vi "SendTriggerCAN.vi"(8 "error in (no error)":errorcluster, 11 "interface object in":refnum<k20>) -> (0 "error out":errorcluster, 3 "interface object out":refnum<k20>)   [LabVIEW 2014]
uses:
  <vilib>/RioEmbeddedCAN/RioEmbeddedCAN.llb/CANFrameControl.ctl
  Global Data.vi
  <vilib>/RioEmbeddedCAN/RioEmbeddedCAN.llb/CANWaitTransmitComplete.vi
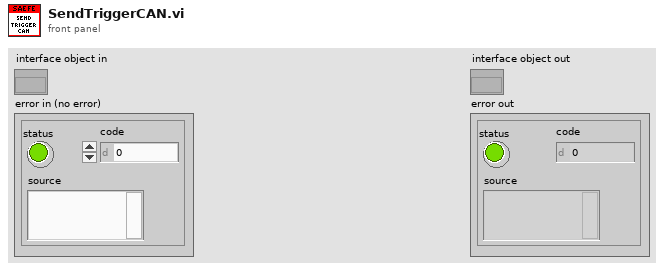
[diagram p1: front panel]
types:
  T1 = typedef "CANFrameControl.ctl" = cluster{"identifier":u32, "extended?":bool, "type":u8, "payload":u8[]}
  T2 = typedef "FPGA Telemetry.ctl" = cluster{"CPU Load":cluster{"Total (%)":dbl, "Time Critical (%)":dbl, "Timed Structures (%)":dbl, "High (%)":dbl, "Above Normal (%)":dbl, "Normal (%)":dbl, "Background (%)":dbl, "Idle (%)":dbl, "ISR (%)":dbl}, "SVehicleStatus":cluster{"BMS Status":T3, "MC Status":T3, "Shutdown Status":T3, "sbRIO Status":T3, "Vehicle Status":T3, "Shutdown State":enum16{"NI.SC.Initial", "NI.SC.History", "NI.SC.ShallowHistory", "NI.SC.Terminal", "Coolant Pump Started/AIR's On", "AIRs On", "Precharge", "TSMS Off"}, "AIR Status":T6, "Remote Return to Pits":bool, "Reason for Shutdown":T7, "MC State Machine Status":enum16{"NI.SC.Initial", "NI.SC.History", "NI.SC.ShallowHistory", "NI.SC.Terminal", "Broadcast Diag", "Let Current Drop then Disable AIR's", "Enabled", "Disabled"}}, "iPhone HF Data":cluster{"gXiPhone":dbl, "gYiPhone":dbl, "gZiPhone":dbl, "nYawXiPhone":dbl, "nYawYiPhone":dbl, "nYawZiPhone":dbl}, "iPhone LF Data":cluster{"nLatiPhone":dbl, "nLongiPhone":dbl, "nGPSiPhone":dbl}, "stop":bool, "VSupplyOffset":fxp<+,12,4>, "VsbRIOSupply":fxp<+/-,25,6>, "bFPGALED":bool, "TSBRIO":fxp<+/-,33,17>, "rTPS2Unscaled":fxp<+/-,16,1>, "rTPS1Unscaled":fxp<+/-,16,1>, "bTPSConsistent":bool, "bTPSInRange":bool, "rThrottle":fxp<+/-,33,22>, "VTPS2":fxp<+/-,24,5>, "rTPS2":fxp<+/-,31,22>, "VTPS1":fxp<+/-,24,5>, "rTPS1":fxp<+/-,31,22>, "rTPS2Max":fxp<+,16,4>, "rTPS2Min":fxp<+,16,4>, "rTPS1Max":fxp<+,16,4>, "rTPS1Min":fxp<+,16,4>, "bCoolantPumpEnable":bool, "bRTDSEnable":bool, "bTSMSInStatus":bool, "bPosAIREnable":bool, "bBMSOK":bool, "bIMDOK":bool, "bBSPDOK":bool, "bSBRIOOK2":bool, "bSBRIOOK1":bool, "bTSMSOutStatus":bool, "eGreenDash":T8, "eYellowDash":T8, "eRedDash":T8, "bMotorControllerEnable":bool, "tCurrentLap":u32, "bNewLap":bool, "tLastLap":u32, "tLapMin":u32, "V5VSupply":fxp<+/-,24,5>, "bWheelRL":bool, "bWheelRR":bool, "bWheelFR":bool, "bWheelFL":bool, "VBrakePressureR":fxp<+/-,24,5>, "VBrakePressureF":fxp<+/-,24,5>, "bWheelRRStopped":bool, "bWheelRLStopped":bool, "bWheelFRStopped":bool, "bWheelFLStopped":bool, "tWheelRLPeriod":u32, "tWheelRRPeriod":u32, "tWheelFRPeriod":u32, "tWheelFLPeriod":u32, "bBrakeLight":bool, "VShockRR":fxp<+/-,24,5>, "VShockRL":fxp<+/-,24,5>, "VShockFR":fxp<+/-,24,5>, "VShockFL":fxp<+/-,24,5>, "IHighCurrent":fxp<+/-,24,15>, "ILowCurrent":fxp<+/-,24,15>, "pBrakeR":fxp<+,26,13>, "pBrakeF":fxp<+,26,13>, "bHighCurrentOK":bool, "bLowCurrentOK":bool, "bBrakeROK":bool, "bBrakeFOK":bool, "VSteerWheelMiddle":fxp<+/-,26,5>, "aSteerWheel":fxp<+/-,31,13>, "nWheelFL":fxp<+/-,32,16>, "nWheelFR":fxp<+/-,32,16>, "nWheelRL":fxp<+/-,32,16>, "nWheelRR":fxp<+/-,32,16>, "ADXL345 Output":T9, "Tire Diameter(m)":fxp<+,16,1>, "vWheelRR":fxp<+/-,32,18>, "vWheelRL":fxp<+/-,32,18>, "vWheelFR":fxp<+/-,32,18>, "vWheelFL":fxp<+/-,32,18>, "vWheelLowest":fxp<+/-,32,18>, "vWheelHighest":fxp<+/-,32,18>, "bAccel":bool, "vAxleF":fxp<+/-,33,19>, "vCar":fxp<+/-,33,19>, "sLap":fxp<+,32,12>, "rSlipRL":fxp<+/-,12,1>, "rSlipRR":fxp<+/-,12,1>, "rSlipFL":fxp<+/-,12,1>, "rSlipFR":fxp<+/-,12,1>, "NLap":u8, "tLapReference":u32, "tFastestLap":u32}
  T3 = typedef "Subsystem Status.ctl" = cluster{"eStatusSeverity":T4, "NValue":sgl, "CMessage":T5, "bNotOK":bool}
  T4 = typedef "Subsystem Status Severity.ctl" = enum16{"Okay", "Short Warning", "Long Warning", "Return to Pits", "Error", "Danger"}
  T5 = typedef "Subsystem Status Message.ctl" = enum16{"ControllerTemperature", "MotorTemperature", "BatteryTemperature", "BatteryLowVoltage", "LVBattery", "sbRIOTemperature", "Precharge", "BSPD", "IMD", "RemoteReturnToPits", "EStopInterrupted", "NoCellComms", "MCOverSpeed", "MCOverCurrent", "MCOverVoltage", "MCInverterOverTemp", "MCDirectionCommand", "MCInverterTimeout", "MCDesatFault", "MCHWOverCurrent", "MCUnderVoltage", "MCCommandMessageLost", "MotorOverTemp", "MCModAOverTemp", "MCModBOverTemp", "MCModCOverTemp", "MCPCBOverTemp", "MCGateDrv1OverTemp", "MCDateDrv2OverTemp", "MCCurrentSensorFault", "MCResolverNotConnected", "ShutdownLatchTripped", "UnknownBMS", "RemoteEmergency"}
  T6 = typedef "AIR Status.ctl" = enum16{"Off", "Precharge", "On"}
  T7 = typedef "Reason for Shutdown.ctl" = enum16{"None", "BMS", "Shutdown", "sbRIO", "MC", "Remote"}
  T8 = typedef "Dash LED Status.ctl" = enum16{"Off", "Flashing", "On"}
  T9 = typedef "ADXL345 Output.ctl" = cluster{"X":fxp<+/-,14,4>, "Y":fxp<+/-,14,4>, "Z":fxp<+/-,14,4>}
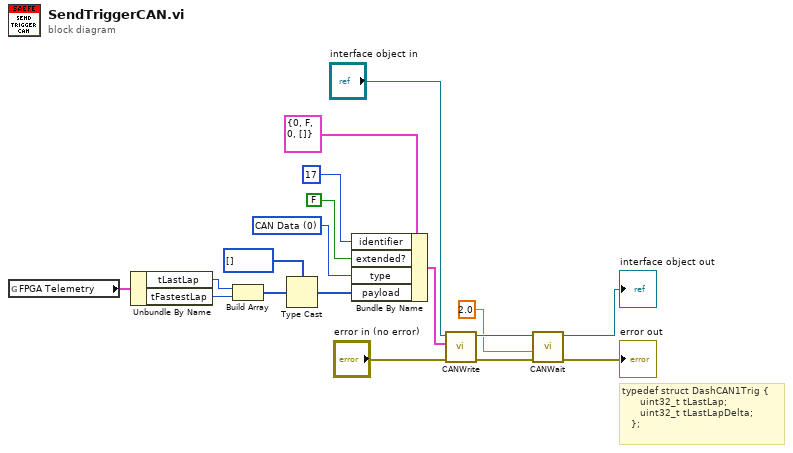
[diagram p0: block diagram]
diagram:
  w10 = u8 0 items=["CAN Data", "CAN Remote"] ("type")
  # "typedef struct DashCAN1Trig {\n      uint32_t tLastLap;\n      uint32_t tLastLapDelta;\n   };"
  n1 = global read "Global Data.vi" "FPGA Telemetry"() -> (w5:T2)
  n2 = Unbundle By Name(w5) -> ("tLastLap"=w4:u32, "tFastestLap"=w3:u32)
  n3 = Build Array(w4, w3) -> (w6:u32[])
  n4 = Type Cast(type=u8[] [], x=w6) -> (*(type *) &x=w8:u8[])
  n5 = Bundle By Name(cluster=T1 {"identifier"=0, "extended?"=FALSE, "type"=0, "payload"=[]} ("CAN frame"), "identifier"=u32 17, "extended?"=FALSE, "type"=w10, "payload"=w8) -> (w15:T1)
  n6 = call <vilib>:"CANWrite.vi"("error in (no error)"="error in (no error)", "CAN frame"=w15, "interface object in"="interface object in") -> ("error out"=w13:errorcluster, "interface object out"=w14:refnum<k20>)  [unwired: 7 in]
  n7 = call-poly <vilib>:"CANWait.vi"("error in (no error)"=w13, "timeout (0 s)"=2.0, "interface object in"=w14) -> ("error out"=→"error out":errorcluster, "interface object out"=→"interface object out":refnum<k20>)  [unwired: 7 in]
